vi "Write to String Log.vi"(10 "String to Log":string, 11 "String Log Sink in":refnum<class "String Log Sink.lvclass">) -> (0 "error out":errorcluster, 3 "String Log Sink out":refnum<class "String Log Sink.lvclass">)   [LabVIEW 2020, in "MVA Framework.lvlib" / "String Log Sink.lvclass"]
uses:
  String Log Sink.lvclass
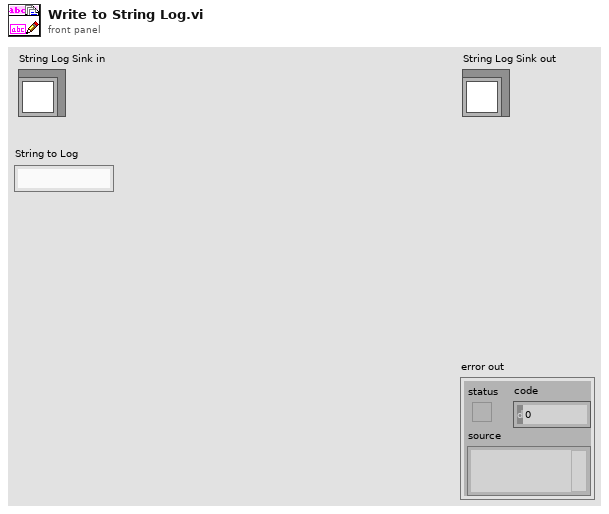
[diagram p1: front panel]
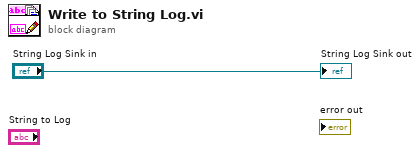
[diagram p0: block diagram]
diagram:
  "String Log Sink out" <- "String Log Sink in"
